vi "EPTx_RT_mul-inj_Final.vi"(0 "EPTxSupervisor_rt":T13={"Sync"=FALSE, "CurrentCAD"=0.0, "MaxCAD"=720.0, "HistoryCAD"=61.0, "CADRate"=0.0, "AvgSpeed"=0.0, "Config"=FALSE, "Rcvg Primary"=FALSE, "Stall"=FALSE, "Overflow"=FALSE, "Ratio Error"=FALSE, "Pattern Error"=FALSE, "Aux Warning"=FALSE, "Watchdog Error"=FALSE}, 1 "PatternConfig":T16 {"Max Rate [Hz]" format="%#_3p"}, 2 "SimulatorConfig":T18={"Sim Speed [RPM]"=1000.0, "Ramp Rate [RPM/s]"=50.0, "Rotations"=2, "Pause"=FALSE, "Pause Angle [CAD]"=0.0, "Max Offset [RPM]"=0.0, "Cylinders"=6}, 5 "EPTxState":T15={"Sync Enable"=TRUE, "Clear Errors"=FALSE, "Sim Enable"=FALSE, "Sim Speed [RPM]"=1000.0}, 7 "EPTxFilters":T14={"Primary [s]"=5e-06, "Aux 1 [s]"=5e-06, "Aux 2 [s]"=0.0, "Aux 3 [s]"=0.0, "Aux 4 [s]"=0.0} {"Aux 4 [s]" format="%#_6p"; "Aux 3 [s]" format="%#_6p"; "Aux 2 [s]" format="%#_6p"; "Aux 1 [s]" format="%#_6p"; "Primary [s]" format="%#_6p"}, 9 "RT_Input":T17={"Load"=FALSE, "History_[CAD]"=63, "Stall_Speed_[RPM]"=200.0, "Delay_time[ms]"=0.0, "DrvMode"=0} caption="簇", 11 "Inj_Timing":T12, 12 "Inj_Duration_in":T11) -> (3 "Config_number":T10 caption="簇", 4 "CylinderSig":T6={"CylinderSig_1"={"Cylinder1_H_R[CAD]"=204.0, "Cylinder1_H_F[CAD]"=210.0}, "CylinderSig_2"={"Cylinder2_H_R[CAD]"=684.0, "Cylinder2_H_F[CAD]"=690.0}, "CylinderSig_3"={"Cylinder3_H_R[CAD]"=444.0, "Cylinder3_H_F[CAD]"=450.0}, "CylinderSig_4"={"Cylinder4_H_R[CAD]"=90.0, "Cylinder4_H_F[CAD]"=100.0}, "CylinderSig_5"={"Cylinder5_H_R[CAD]"=324.0, "Cylinder5_H_F[CAD]"=330.0}, "CylinderSig_6"={"Cylinder6_H_R[CAD]"=0.0, "Cylinder6_H_F[CAD]"=0.0}} caption="簇", 6 "EPTxPatternConfig":T4 {"Pattern"."Aux 4" format="%#_16g"; "Pattern"."Aux 3" format="%#_16g"; "Pattern"."Aux 2" format="%#_16g"; "Pattern"."Aux 1" format="%#_16g"; "Pattern"."Primary" format="%#_16g"}, 8 "Tick_output":T1, 10 "EPTxControl":T3={"Sync Enable"=FALSE, "Clear Errors"=FALSE, "Sim Enable"=FALSE, "Sim Rate"=63.999996185302734, "Watchdog"=FALSE}, 13 "Cmd_Seq":T19, 14 "Lighting":T7 caption="簇", 15 "EPTxData":T2={"Sync"=TRUE, "CurrentCAD"=122.91406, "Speed [RPM]"=999.75, "Config"=FALSE, "Rcvg Primary"=TRUE, "Stall"=FALSE, "Overflow"=FALSE, "Ratio Error"=FALSE, "Pattern Error"=FALSE, "Aux Warning"=FALSE, "Watchdog Error"=FALSE})   [LabVIEW 2023]
uses:
  <vilib>/Powertrain Controls/Device Drivers/Engine Position Tracking/EPTx/RevA/RT/Controls/Simulator Config.ctl
  <vilib>/Powertrain Controls/Device Drivers/Engine Position Tracking/EPTx/RevA/RT/Controls/Pattern Config.ctl
  <vilib>/Powertrain Controls/Device Drivers/Engine Position Tracking/EPTx/RevA/RT/Controls/EPTxState.ctl
  <vilib>/Powertrain Controls/Device Drivers/Engine Position Tracking/EPTx/RevA/RT/Controls/EPTxFilters.ctl
  <vilib>/Powertrain Controls/Device Drivers/Engine Position Tracking/EPTx/RevA/FPGA/Controls/EPTxSupervisor.ctl
  <vilib>/Powertrain Controls/Device Drivers/Engine Position Tracking/EPTx/RevA/FPGA/Controls/EPTxConfig.ctl
  <vilib>/Powertrain Controls/Device Drivers/Engine Position Tracking/EPTx/RevA/FPGA/Controls/EPTxSimulatorConfig.ctl
  <vilib>/Powertrain Controls/Device Drivers/Engine Position Tracking/EPTx/RevA/FPGA/Controls/EPTxPatternConfig.ctl
  <vilib>/Powertrain Controls/Device Drivers/Engine Position Tracking/EPTx/RevA/FPGA/Controls/Patterns.ctl
  <vilib>/Powertrain Controls/Device Drivers/Engine Position Tracking/EPTx/RevA/FPGA/Controls/EPTxControl.ctl
  <vilib>/Powertrain Controls/Device Drivers/Engine Position Tracking/EPTx/RevA/RT/Controls/EPTxData.ctl
  <vilib>/Powertrain Controls/Device Drivers/Engine Position Tracking/EPTx/RevA/RT/Controls/EPTxPattern.ctl
  <vilib>/Powertrain Controls/Device Drivers/Engine Position Tracking/EPTx/RevA/RT/Controls/Pattern.ctl
  <vilib>/Powertrain Controls/Device Drivers/Engine Position Tracking/EPTx/RevA/RT/Controls/EPTxSettings.ctl
  <vilib>/Powertrain Controls/Device Drivers/Engine Position Tracking/EPTx/RevA/RT/Controls/Settings - Tooth.ctl
  <vilib>/Powertrain Controls/Device Drivers/Engine Position Tracking/EPTx/RevA/RT/Controls/Direction Detection.ctl
  <vilib>/Powertrain Controls/Device Drivers/Engine Position Tracking/EPTx/RevA/RT/Controls/Settings - Pattern.ctl
  <vilib>/Powertrain Controls/Device Drivers/Engine Position Tracking/EPTx/RevA/RT/Controls/Settings - Token.ctl
  <vilib>/Powertrain Controls/Device Drivers/Engine Position Tracking/EPTx/RevA/RT/Controls/Aux Signal.ctl
  <vilib>/Powertrain Controls/Device Drivers/Engine Position Tracking/EPTx/RevA/RT/Controls/Aux Type.ctl
  <vilib>/Powertrain Controls/Device Drivers/Engine Position Tracking/EPTx/RevA/RT/Controls/Aux Threshold.ctl
  <vilib>/Powertrain Controls/Device Drivers/Engine Position Tracking/EPTx/RevA/RT/EPTx - RevA - RT.lvlib
  <vilib>/Powertrain Controls/Device Drivers/Engine Position Tracking/EPTx/RevA/FPGA/EPTx - RevA - FPGA.lvlib
panel:
  out "CAD":sgl
  out "AvgSpeed":fxp<+,17,15>
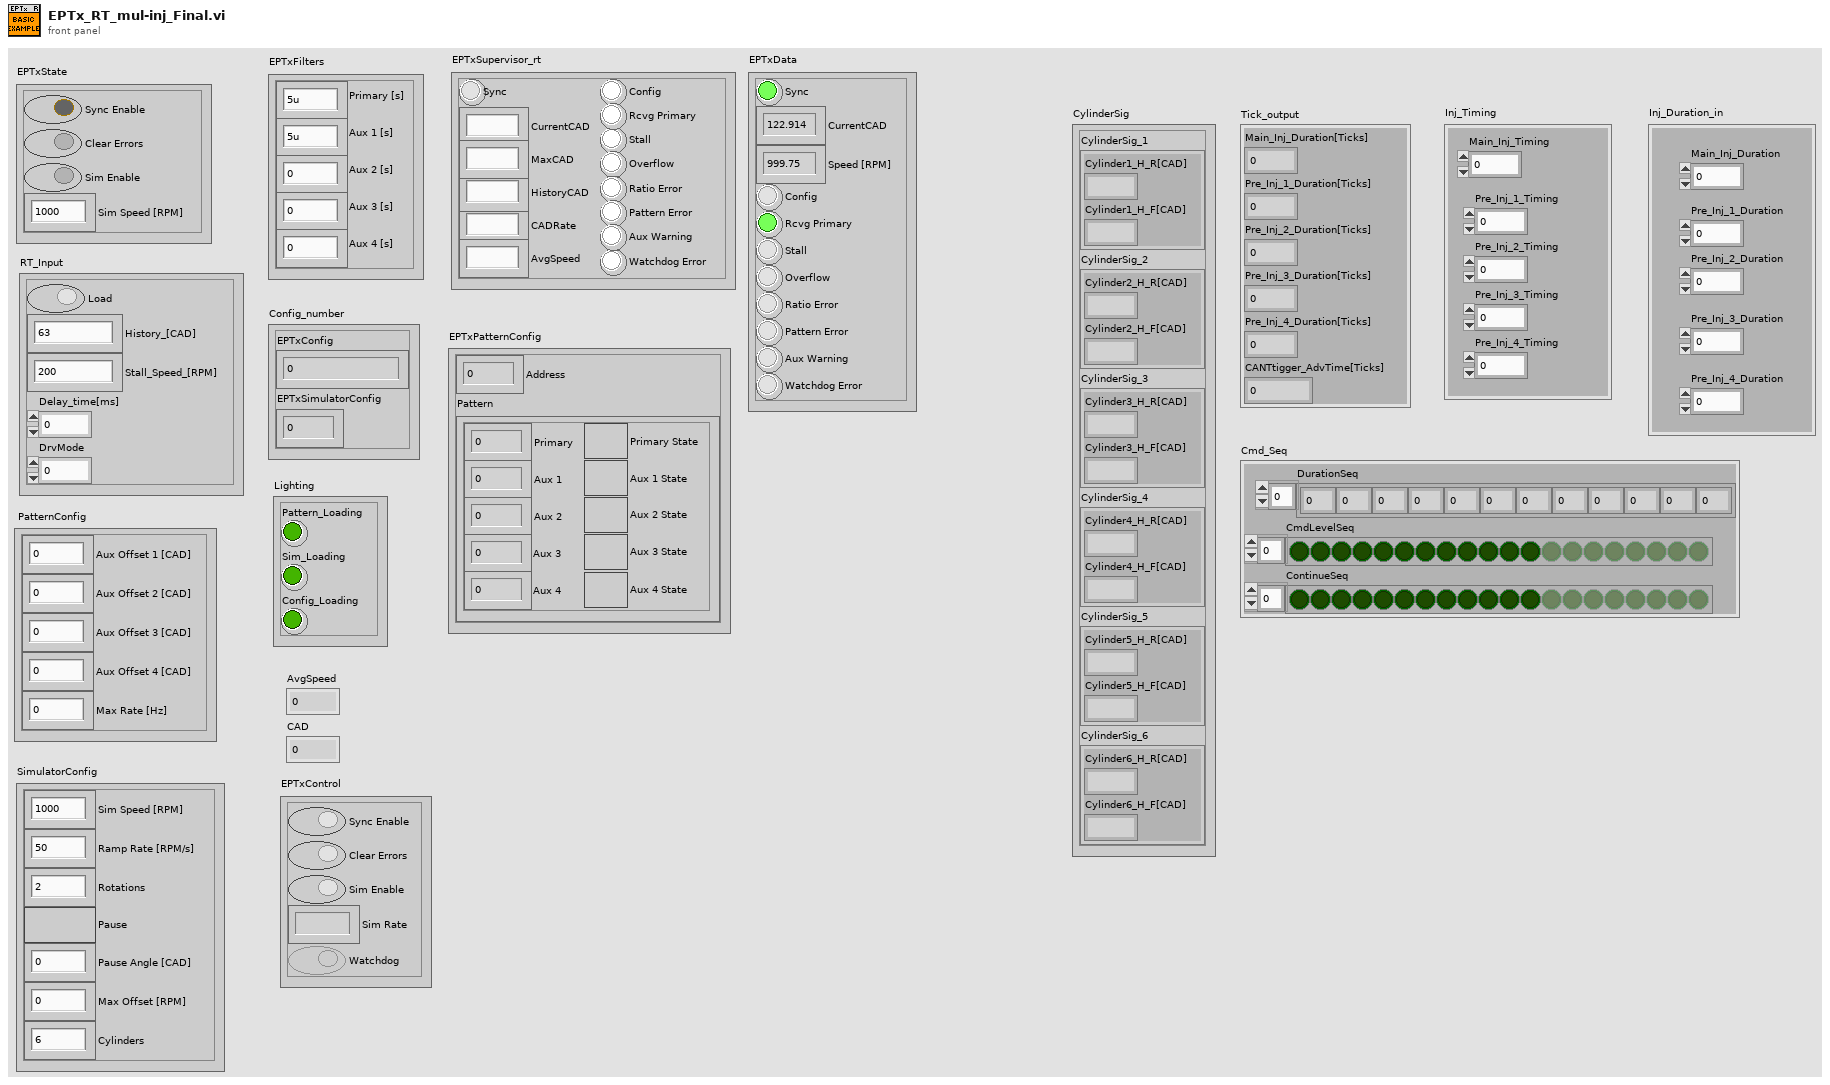
[diagram p1: front panel]
types:
  T1 = cluster{"Main_Inj_Duration[Ticks]":u32, "Pre_Inj_1_Duration[Ticks]":u32, "Pre_Inj_2_Duration[Ticks]":u32, "Pre_Inj_3_Duration[Ticks]":u32, "Pre_Inj_4_Duration[Ticks]":u32, "CANTtigger_AdvTime[Ticks]":u32}
  T2 = typedef "EPTx - RevA - RT.lvlib/EPTxData.ctl" = cluster{"Sync":bool, "CurrentCAD":sgl, "Speed [RPM]":sgl, "Config":bool, "Rcvg Primary":bool, "Stall":bool, "Overflow":bool, "Ratio Error":bool, "Pattern Error":bool, "Aux Warning":bool, "Watchdog Error":bool}
  T3 = typedef "EPTx - RevA - FPGA.lvlib/EPTxControl.ctl" = cluster{"Sync Enable":bool, "Clear Errors":bool, "Sim Enable":bool, "Sim Rate":fxp<+,24,6>, "Watchdog":bool}
  T4 = typedef "EPTx - RevA - FPGA.lvlib/EPTxPatternConfig.ctl" = cluster{"Address":fxp<+,14,14>, "Pattern":T5}
  T5 = typedef "EPTx - RevA - FPGA.lvlib/Patterns.ctl" = cluster{"Primary":fxp<+,19,12>, "Primary State":bool, "Aux 1":fxp<+,19,12>, "Aux 1 State":bool, "Aux 2":fxp<+,19,12>, "Aux 2 State":bool, "Aux 3":fxp<+,19,12>, "Aux 3 State":bool, "Aux 4":fxp<+,19,12>, "Aux 4 State":bool}
  T6 = cluster{"CylinderSig_1":cluster{"Cylinder1_H_R[CAD]":fxp<+,18,11>, "Cylinder1_H_F[CAD]":fxp<+,18,11>}, "CylinderSig_2":cluster{"Cylinder2_H_R[CAD]":fxp<+,18,11>, "Cylinder2_H_F[CAD]":fxp<+,18,11>}, "CylinderSig_3":cluster{"Cylinder3_H_R[CAD]":fxp<+,18,11>, "Cylinder3_H_F[CAD]":fxp<+,18,11>}, "CylinderSig_4":cluster{"Cylinder4_H_R[CAD]":fxp<+,18,11>, "Cylinder4_H_F[CAD]":fxp<+,18,11>}, "CylinderSig_5":cluster{"Cylinder5_H_R[CAD]":fxp<+,18,11>, "Cylinder5_H_F[CAD]":fxp<+,18,11>}, "CylinderSig_6":cluster{"Cylinder6_H_R[CAD]":fxp<+,18,11>, "Cylinder6_H_F[CAD]":fxp<+,18,11>}}
  T7 = cluster{"Pattern_Loading":bool, "Sim_Loading":bool, "Config_Loading":bool}
  T8 = typedef "EPTx - RevA - FPGA.lvlib/EPTxConfig.ctl" = u64
  T9 = typedef "EPTx - RevA - FPGA.lvlib/EPTxSimulatorConfig.ctl" = u32
  T10 = cluster{"EPTxConfig":T8, "EPTxSimulatorConfig":T9}
  T11 = cluster{"Main_Inj_Duration":sgl, "Pre_Inj_1_Duration":sgl, "Pre_Inj_2_Duration":sgl, "Pre_Inj_3_Duration":sgl, "Pre_Inj_4_Duration":sgl}
  T12 = cluster{"Main_Inj_Timing":sgl, "Pre_Inj_1_Timing":sgl, "Pre_Inj_2_Timing":sgl, "Pre_Inj_3_Timing":sgl, "Pre_Inj_4_Timing":sgl}
  T13 = typedef "EPTx - RevA - FPGA.lvlib/EPTxSupervisor.ctl" = cluster{"Sync":bool, "CurrentCAD":fxp<+,18,11>, "MaxCAD":fxp<+,11,11>, "HistoryCAD":fxp<+,11,11>, "CADRate":fxp<+,22,8>, "AvgSpeed":fxp<+,17,15>, "Config":bool, "Rcvg Primary":bool, "Stall":bool, "Overflow":bool, "Ratio Error":bool, "Pattern Error":bool, "Aux Warning":bool, "Watchdog Error":bool}
  T14 = typedef "EPTx - RevA - RT.lvlib/EPTxFilters.ctl" = cluster{"Primary [s]":sgl, "Aux 1 [s]":sgl, "Aux 2 [s]":sgl, "Aux 3 [s]":sgl, "Aux 4 [s]":sgl}
  T15 = typedef "EPTx - RevA - RT.lvlib/EPTxState.ctl" = cluster{"Sync Enable":bool, "Clear Errors":bool, "Sim Enable":bool, "Sim Speed [RPM]":sgl}
  T16 = typedef "EPTx - RevA - RT.lvlib/Pattern Config.ctl" = cluster{"Aux Offset 1 [CAD]":sgl, "Aux Offset 2 [CAD]":sgl, "Aux Offset 3 [CAD]":sgl, "Aux Offset 4 [CAD]":sgl, "Max Rate [Hz]":sgl}
  T17 = cluster{"Load":bool, "History_[CAD]":u8, "Stall_Speed_[RPM]":sgl, "Delay_time[ms]":sgl, "DrvMode":u32}
  T18 = typedef "EPTx - RevA - RT.lvlib/Simulator Config.ctl" = cluster{"Sim Speed [RPM]":sgl, "Ramp Rate [RPM/s]":sgl, "Rotations":u8, "Pause":bool, "Pause Angle [CAD]":sgl, "Max Offset [RPM]":sgl, "Cylinders":u8}
  T19 = cluster{"DurationSeq":u32[], "CmdLevelSeq":bool[], "ContinueSeq":bool[]}
  T20 = cluster{"Duration1":sgl, "Duratiion2":sgl, "Duration3":sgl, "Duration4":sgl, "Duration5":sgl, "Duration6":sgl, "Duration7":sgl, "Duration8":sgl, "Duration9":sgl, "Duration10":sgl, "Duration11":sgl, "Duration12":sgl}
  T21 = cluster{"CylinderSig_1":cluster{"Cylinder1_H_R [CAD]":fxp<+,18,11>, "Cylinder1_H_F [CAD]":fxp<+,18,11>}, "CylinderSig_2":cluster{"Cylinder2_H_R [CAD]":fxp<+,18,11>, "Cylinder2_H_F [CAD]":fxp<+,18,11>}, "CylinderSig_3":cluster{"Cylinder3_H_R [CAD]":fxp<+,18,11>, "Cylinder3_H_F [CAD]":fxp<+,18,11>}, "CylinderSig_4":cluster{"Cylinder4_H_R [CAD]":fxp<+,18,11>, "Cylinder4_H_F [CAD]":fxp<+,18,11>}, "CylinderSig_5":cluster{"Cylinder5_H_R [CAD]":fxp<+,18,11>, "Cylinder5_H_F [CAD]":fxp<+,18,11>}, "CylinderSig_6":cluster{"Cylinder6_H_R [CAD]":fxp<+,18,11>, "Cylinder6_H_F [CAD]":fxp<+,18,11>}}
  T22 = cluster{"Cylinder6_H_R [CAD]":fxp<+,18,11>, "Cylinder6_H_F [CAD]":fxp<+,18,11>}
  T23 = cluster{"Cylinder5_H_R [CAD]":fxp<+,18,11>, "Cylinder5_H_F [CAD]":fxp<+,18,11>}
  T24 = cluster{"Cylinder4_H_R [CAD]":fxp<+,18,11>, "Cylinder4_H_F [CAD]":fxp<+,18,11>}
  T25 = cluster{"Cylinder3_H_R [CAD]":fxp<+,18,11>, "Cylinder3_H_F [CAD]":fxp<+,18,11>}
  T26 = cluster{"Cylinder2_H_R [CAD]":fxp<+,18,11>, "Cylinder2_H_F [CAD]":fxp<+,18,11>}
  T27 = cluster{"Cylinder1_H_R [CAD]":fxp<+,18,11>, "Cylinder1_H_F [CAD]":fxp<+,18,11>}
  T28 = cluster{"Pattern Loading":bool, "Sim Loading":bool, "Config Loading":bool}
  T29 = typedef "EPTx - RevA - RT.lvlib/EPTxSettings.ctl" = cluster{"Rotation":u8, "Ratios":sgl[], "Thresholds":sgl[], "Tooth":T30, "Pattern":T32[], "Token":T33[], "Aux Threshold Min":T36, "Aux Threshold Max":T36}
  T30 = typedef "EPTx - RevA - RT.lvlib/Settings - Tooth.ctl" = cluster{"Rising Edge":bool, "Falling Edge":bool, "Direction\nDetection":T31, "Level":bool, "Parameter":sgl}
  T31 = typedef "EPTx - RevA - RT.lvlib/Direction Detection.ctl" = enum16{"None", "Aux Signal", "Length"}
  T32 = typedef "EPTx - RevA - RT.lvlib/Settings - Pattern.ctl" = cluster{"Ratio Index":u8, "Ratio Count":u16, "Angle":sgl, "dAngle":sgl}
  T33 = typedef "EPTx - RevA - RT.lvlib/Settings - Token.ctl" = cluster{"Length":u16, "Start Index":u8, "Start Count":u16, "Aux 1":T34, "Aux 1 Type":T35, "Aux 1 Max":u16, "Aux 1 Min":u16, "Aux 2":T34, "Aux 2 Type":T35, "Aux 2 Max":u16, "Aux 2 Min":u16, "End Index":u8, "End Count":u16}
  T34 = typedef "EPTx - RevA - RT.lvlib/Aux Signal.ctl" = enum8{"---", "Aux 1", "Aux 2", "Aux 3", "Aux 4"}
  T35 = typedef "EPTx - RevA - RT.lvlib/Aux Type.ctl" = enum8{"Falling", "Rising", "Low", "High", "Ratio"}
  T36 = typedef "EPTx - RevA - RT.lvlib/Aux Threshold.ctl" = cluster{"Aux 1":sgl, "Aux 2":sgl, "Aux 3":sgl, "Aux 4":sgl}
  T37 = typedef "EPTx - RevA - RT.lvlib/EPTxPattern.ctl" = cluster{"Rotations":u8, "Cylinders":u8, "Primary":T38[], "Aux 1":T38[], "Aux 2":T38[], "Aux 3":T38[], "Aux 4":T38[]}
  T38 = typedef "EPTx - RevA - RT.lvlib/Pattern.ctl" = cluster{"Angle":sgl, "State":bool}
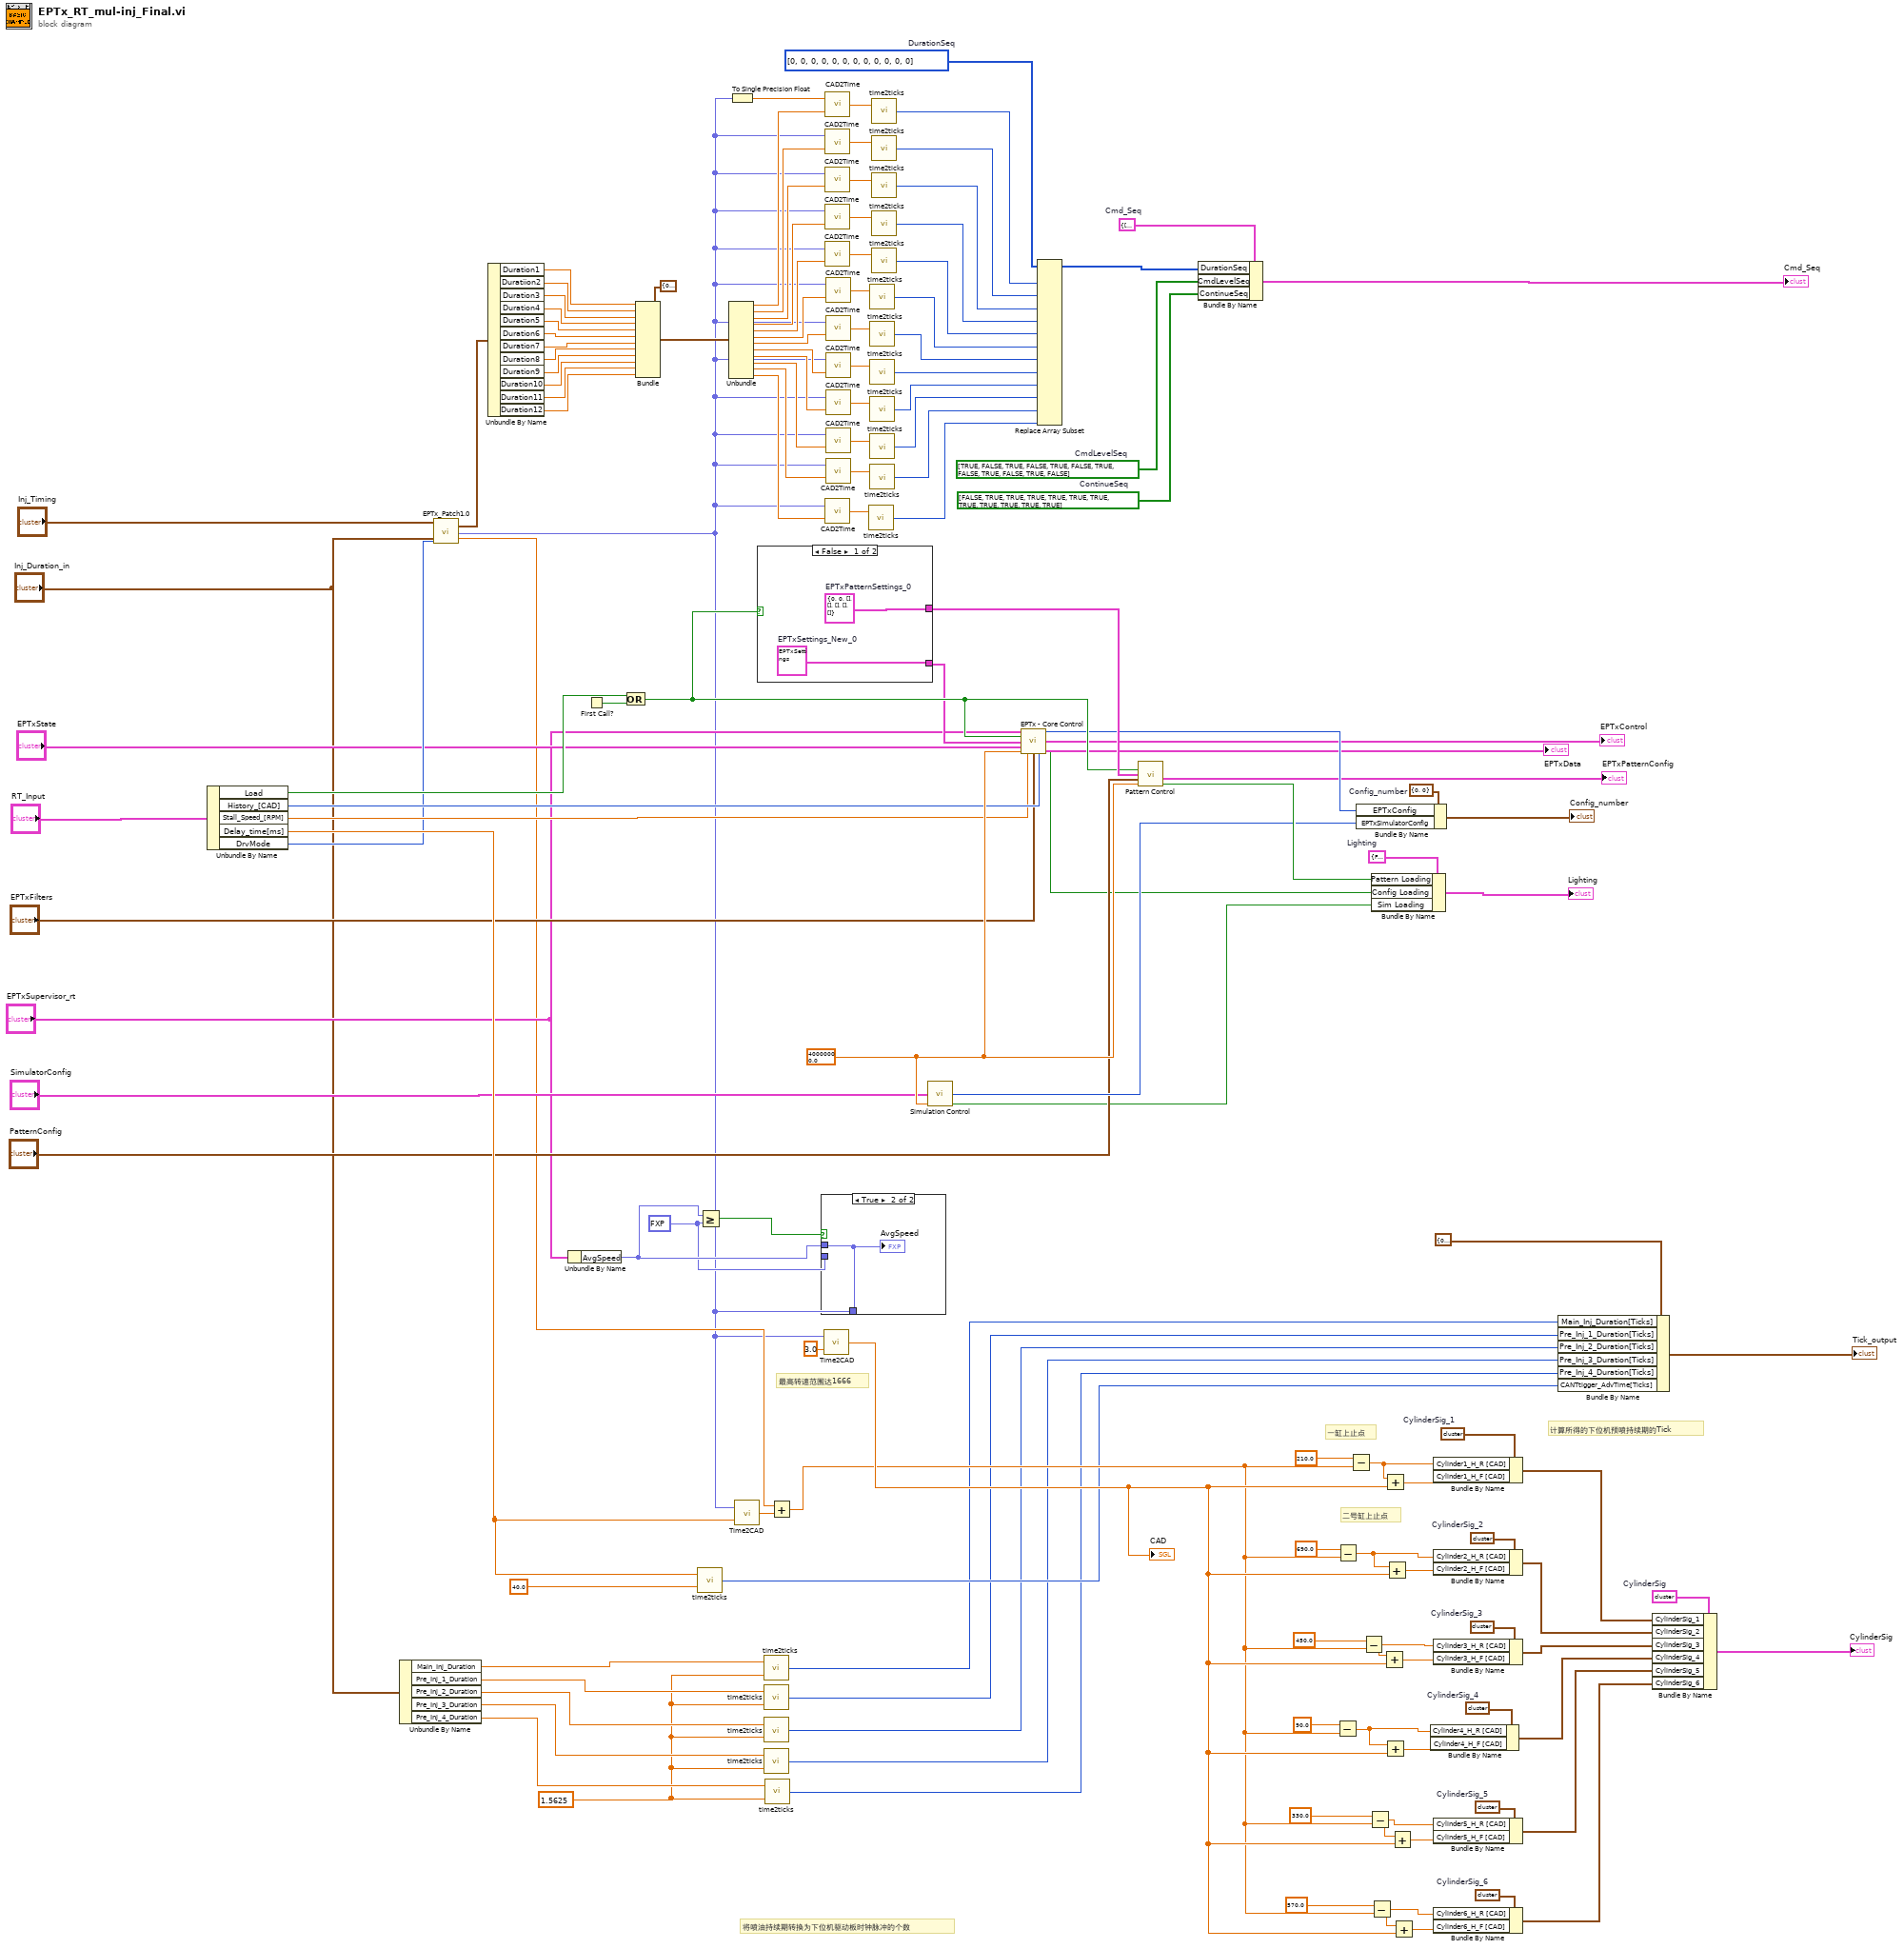
[diagram p0: block diagram]
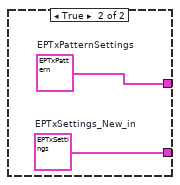
[diagram p3: hidden frame]
diagram:
  w6 = bool[] [TRUE, FALSE, TRUE, FALSE, TRUE, FALSE, TRUE, FALSE, TRUE, FALSE, TRUE, FALSE]  # CmdLevelSeq
  w7 = bool[] [FALSE, TRUE, TRUE, TRUE, TRUE, TRUE, TRUE, TRUE, TRUE, TRUE, TRUE, TRUE]  # ContinueSeq
  w8 = fxp<+,7,8> 250.0 ("y")
  w96 = T19 {"DurationSeq"=[0, 0, 0, 0, 0, 0, 0, 0, 0, 0, 0, 0], "CmdLevelSeq"=[FALSE, FALSE, FALSE, FALSE, FALSE, FALSE, FALSE, FALSE, FALSE, FALSE, FALSE, FALSE], "ContinueSeq"=[FALSE, FALSE, FALSE, FALSE, FALSE, FALSE, FALSE, FALSE, FALSE, FALSE, FALSE, FALSE]}  # Cmd_Seq
  w80 = u32[] [0, 0, 0, 0, 0, 0, 0, 0, 0, 0, 0, 0]  # DurationSeq
  w10 = sgl 1.5625 ("y")
  w111 = T21 {"CylinderSig_1"={"Cylinder1_H_R [CAD]"=204.0, "Cylinder1_H_F [CAD]"=210.0}, "CylinderSig_2"={"Cylinder2_H_R [CAD]"=684.0, "Cylinder2_H_F [CAD]"=690.0}, "CylinderSig_3"={"Cylinder3_H_R [CAD]"=444.0, "Cylinder3_H_F [CAD]"=450.0}, "CylinderSig_4"={"Cylinder4_H_R [CAD]"=90.0, "Cylinder4_H_F [CAD]"=100.0}, "CylinderSig_5"={"Cylinder5_H_R [CAD]"=324.0, "Cylinder5_H_F [CAD]"=330.0}, "CylinderSig_6"={"Cylinder6_H_R [CAD]"=0.0, "Cylinder6_H_F [CAD]"=0.0}}  # CylinderSig
  w128 = T22 {"Cylinder6_H_R [CAD]"=0.0, "Cylinder6_H_F [CAD]"=0.0}  # CylinderSig_6
  w129 = T23 {"Cylinder5_H_R [CAD]"=324.0, "Cylinder5_H_F [CAD]"=330.0}  # CylinderSig_5
  w130 = T24 {"Cylinder4_H_R [CAD]"=90.0, "Cylinder4_H_F [CAD]"=100.0}  # CylinderSig_4
  w131 = T25 {"Cylinder3_H_R [CAD]"=444.0, "Cylinder3_H_F [CAD]"=450.0}  # CylinderSig_3
  w132 = T26 {"Cylinder2_H_R [CAD]"=684.0, "Cylinder2_H_F [CAD]"=690.0}  # CylinderSig_2
  w133 = T27 {"Cylinder1_H_R [CAD]"=204.0, "Cylinder1_H_F [CAD]"=210.0}  # CylinderSig_1
  w138 = T10 {"EPTxConfig"=0, "EPTxSimulatorConfig"=0}  # Config_number
  w140 = T28 {"Pattern Loading"=FALSE, "Sim Loading"=FALSE, "Config Loading"=FALSE}  # Lighting
  w144 = sgl 40000000.0 ("Frequency (40M) [Hz]")
  # "最高转速范围达1666"
  # "计算所得的下位机预喷持续期的Tick"
  # "二号缸上止点"
  # "一缸上止点"
  # "将喷油持续期转换为下位机驱动板时钟脉冲的个数"
  n1 = Unbundle By Name("RT_Input") -> ("Load"=w136:bool, "History_[CAD]"=w135:u8, "Stall_Speed_[RPM]"=w134:sgl, "Delay_time[ms]"=w98:sgl, "DrvMode"=w28:u32)
  n2 = Unbundle By Name("Inj_Duration_in") -> ("Main_Inj_Duration"=w36:sgl, "Pre_Inj_1_Duration"=w35:sgl, "Pre_Inj_2_Duration"=w34:sgl, "Pre_Inj_3_Duration"=w33:sgl, "Pre_Inj_4_Duration"=w32:sgl)
  n3 = Unbundle By Name("EPTxSupervisor_rt") -> ("AvgSpeed"=w15:fxp<+,17,15>)
  n4 = First Call?() -> (First Call?: T/F=w142:bool)
  n5 = Compound Arithmetic op=OR ("复合运算")(w136, w142) -> (w141:bool)
  n6 = call <vilib>:"time2ticks.vi"("Clock Frequency (MHz, 40)"=sgl 40.0, "Time (msec)"=w98) -> ("Ticks"=w42:u32)
  n7 = Greater Or Equal?(x=w15, y=w8) -> (x >= y?=w16:bool)
  n8 = case shown="False" w141 {
    tunnel: [w146 w148] -> w143
    tunnel: [w145 w147] -> w101
    frame False {
      w145 = T29 {"Rotation"=0, "Ratios"=[], "Thresholds"=[], "Tooth"={"Rising Edge"=FALSE, "Falling Edge"=FALSE, "Direction\nDetection"=enum."None", "Level"=FALSE, "Parameter"=0.0}, "Pattern"=[], "Token"=[], "Aux Threshold Min"={"Aux 1"=0.0, "Aux 2"=0.0, "Aux 3"=0.0, "Aux 4"=0.0}, "Aux Threshold Max"={"Aux 1"=0.0, "Aux 2"=0.0, "Aux 3"=0.0, "Aux 4"=0.0}}  # EPTxSettings_New_0
      w146 = T37 {"Rotations"=0, "Cylinders"=0, "Primary"=[], "Aux 1"=[], "Aux 2"=[], "Aux 3"=[], "Aux 4"=[]}  # EPTxPatternSettings_0
    }
    frame True {
      w147 = T29 {"Rotation"=2, "Ratios"=[0.33333334, 1.0, 3.0], "Thresholds"=[0.16666667, 0.6666667, 0.6666667, 2.0, 2.0, 4.0, 999.0], "Tooth"={"Rising Edge"=TRUE, "Falling Edge"=FALSE, "Direction\nDetection"=enum."None", "Level"=FALSE, "Parameter"=0.0}, "Pattern"=[{"Ratio Index"=0, "Ratio Count"=1, "Angle"=0.0, "dAngle"=6.0}, {"Ratio Index"=1, "Ratio Count"=56, "Angle"=6.0, "dAngle"=6.0}, {"Ratio Index"=2, "Ratio Count"=1, "Angle"=342.0, "dAngle"=18.0}, {"Ratio Index"=0, "Ratio Count"=1, "Angle"=360.0, "dAngle"=6.0}, {"Ratio Index"=1, "Ratio Count"=56, "Angle"=366.0, "dAngle"=6.0}, {"Ratio Index"=2, "Ratio Count"=1, "Angle"=702.0, "dAngle"=18.0}], "Token"=[{"Length"=1, "Start Index"=5, "Start Count"=0, "Aux 1"=enum."---", "Aux 1 Type"=enum."Falling", "Aux 1 Max"=0, "Aux 1 Min"=0, "Aux 2"=enum."Aux 2", "Aux 2 Type"=enum."Ratio", "Aux 2 Max"=73, "Aux 2 Min"=73, "End Index"=0, "End Count"=0}], "Aux Threshold Min"={"Aux 1"=1.8809524, "Aux 2"=1.2142857, "Aux 3"=0.0, "Aux 4"=0.0}, "Aux Threshold Max"={"Aux 1"=2.7857144, "Aux 2"=1.8809524, "Aux 3"=999.0, "Aux 4"=999.0}}  # EPTxSettings_New_in
      w148 = T37 {"Rotations"=2, "Cylinders"=6, "Primary"=[{"Angle"=0.0, "State"=FALSE}, {"Angle"=3.0, "State"=TRUE}, {"Angle"=6.0, "State"=FALSE}, {"Angle"=9.0, "State"=TRUE}, {"Angle"=12.0, "State"=FALSE}, {"Angle"=15.0, "State"=TRUE}, {"Angle"=18.0, "State"=FALSE}, {"Angle"=21.0, "State"=TRUE}, {"Angle"=24.0, "State"=FALSE}, {"Angle"=27.0, "State"=TRUE}, {"Angle"=30.0, "State"=FALSE}, {"Angle"=33.0, "State"=TRUE}, {"Angle"=36.0, "State"=FALSE}, {"Angle"=39.0, "State"=TRUE}, {"Angle"=42.0, "State"=FALSE}, {"Angle"=45.0, "State"=TRUE}, {"Angle"=48.0, "State"=FALSE}, {"Angle"=51.0, "State"=TRUE}, {"Angle"=54.0, "State"=FALSE}, {"Angle"=57.0, "State"=TRUE}, {"Angle"=60.0, "State"=FALSE}, {"Angle"=63.0, "State"=TRUE}, {"Angle"=66.0, "State"=FALSE}, {"Angle"=69.0, "State"=TRUE}, {"Angle"=72.0, "State"=FALSE}, {"Angle"=75.0, "State"=TRUE}, {"Angle"=78.0, "State"=FALSE}, {"Angle"=81.0, "State"=TRUE}, {"Angle"=84.0, "State"=FALSE}, {"Angle"=87.0, "State"=TRUE}, {"Angle"=90.0, "State"=FALSE}, {"Angle"=93.0, "State"=TRUE}, {"Angle"=96.0, "State"=FALSE}, {"Angle"=99.0, "State"=TRUE}, {"Angle"=102.0, "State"=FALSE}, {"Angle"=105.0, "State"=TRUE}, {"Angle"=108.0, "State"=FALSE}, {"Angle"=111.0, "State"=TRUE}, {"Angle"=114.0, "State"=FALSE}, {"Angle"=117.0, "State"=TRUE}, {"Angle"=120.0, "State"=FALSE}, {"Angle"=123.0, "State"=TRUE}, {"Angle"=126.0, "State"=FALSE}, {"Angle"=129.0, "State"=TRUE}, {"Angle"=132.0, "State"=FALSE}, {"Angle"=135.0, "State"=TRUE}, {"Angle"=138.0, "State"=FALSE}, {"Angle"=141.0, "State"=TRUE}, {"Angle"=144.0, "State"=FALSE}, {"Angle"=147.0, "State"=TRUE}, {"Angle"=150.0, "State"=FALSE}, {"Angle"=153.0, "State"=TRUE}, {"Angle"=156.0, "State"=FALSE}, {"Angle"=159.0, "State"=TRUE}, {"Angle"=162.0, "State"=FALSE}, {"Angle"=165.0, "State"=TRUE}, {"Angle"=168.0, "State"=FALSE}, {"Angle"=171.0, "State"=TRUE}, {"Angle"=174.0, "State"=FALSE}, {"Angle"=177.0, "State"=TRUE}, {"Angle"=180.0, "State"=FALSE}, {"Angle"=183.0, "State"=TRUE}, {"Angle"=186.0, "State"=FALSE}, {"Angle"=189.0, "State"=TRUE}, {"Angle"=192.0, "State"=FALSE}, {"Angle"=195.0, "State"=TRUE}, {"Angle"=198.0, "State"=FALSE}, {"Angle"=201.0, "State"=TRUE}, {"Angle"=204.0, "State"=FALSE}, {"Angle"=207.0, "State"=TRUE}, {"Angle"=210.0, "State"=FALSE}, {"Angle"=213.0, "State"=TRUE}, {"Angle"=216.0, "State"=FALSE}, {"Angle"=219.0, "State"=TRUE}, {"Angle"=222.0, "State"=FALSE}, {"Angle"=225.0, "State"=TRUE}, {"Angle"=228.0, "State"=FALSE}, {"Angle"=231.0, "State"=TRUE}, {"Angle"=234.0, "State"=FALSE}, {"Angle"=237.0, "State"=TRUE}, {"Angle"=240.0, "State"=FALSE}, {"Angle"=243.0, "State"=TRUE}, {"Angle"=246.0, "State"=FALSE}, {"Angle"=249.0, "State"=TRUE}, {"Angle"=252.0, "State"=FALSE}, {"Angle"=255.0, "State"=TRUE}, {"Angle"=258.0, "State"=FALSE}, {"Angle"=261.0, "State"=TRUE}, {"Angle"=264.0, "State"=FALSE}, {"Angle"=267.0, "State"=TRUE}, {"Angle"=270.0, "State"=FALSE}, {"Angle"=273.0, "State"=TRUE}, {"Angle"=276.0, "State"=FALSE}, {"Angle"=279.0, "State"=TRUE}, {"Angle"=282.0, "State"=FALSE}, {"Angle"=285.0, "State"=TRUE}, {"Angle"=288.0, "State"=FALSE}, {"Angle"=291.0, "State"=TRUE}, {"Angle"=294.0, "State"=FALSE}, {"Angle"=297.0, "State"=TRUE}, {"Angle"=300.0, "State"=FALSE}, {"Angle"=303.0, "State"=TRUE}, {"Angle"=306.0, "State"=FALSE}, {"Angle"=309.0, "State"=TRUE}, {"Angle"=312.0, "State"=FALSE}, {"Angle"=315.0, "State"=TRUE}, {"Angle"=318.0, "State"=FALSE}, {"Angle"=321.0, "State"=TRUE}, {"Angle"=324.0, "State"=FALSE}, {"Angle"=327.0, "State"=TRUE}, {"Angle"=330.0, "State"=FALSE}, {"Angle"=333.0, "State"=TRUE}, {"Angle"=336.0, "State"=FALSE}, {"Angle"=339.0, "State"=TRUE}, {"Angle"=342.0, "State"=FALSE}, {"Angle"=345.0, "State"=TRUE}, {"Angle"=360.0, "State"=FALSE}, {"Angle"=363.0, "State"=TRUE}, {"Angle"=366.0, "State"=FALSE}, {"Angle"=369.0, "State"=TRUE}, {"Angle"=372.0, "State"=FALSE}, {"Angle"=375.0, "State"=TRUE}, {"Angle"=378.0, "State"=FALSE}, {"Angle"=381.0, "State"=TRUE}, {"Angle"=384.0, "State"=FALSE}, {"Angle"=387.0, "State"=TRUE}, {"Angle"=390.0, "State"=FALSE}, {"Angle"=393.0, "State"=TRUE}, {"Angle"=396.0, "State"=FALSE}, {"Angle"=399.0, "State"=TRUE}, {"Angle"=402.0, "State"=FALSE}, {"Angle"=405.0, "State"=TRUE}, {"Angle"=408.0, "State"=FALSE}, {"Angle"=411.0, "State"=TRUE}, {"Angle"=414.0, "State"=FALSE}, {"Angle"=417.0, "State"=TRUE}, {"Angle"=420.0, "State"=FALSE}, {"Angle"=423.0, "State"=TRUE}, {"Angle"=426.0, "State"=FALSE}, {"Angle"=429.0, "State"=TRUE}, {"Angle"=432.0, "State"=FALSE}, {"Angle"=435.0, "State"=TRUE}, {"Angle"=438.0, "State"=FALSE}, {"Angle"=441.0, "State"=TRUE}, {"Angle"=444.0, "State"=FALSE}, {"Angle"=447.0, "State"=TRUE}, {"Angle"=450.0, "State"=FALSE}, {"Angle"=453.0, "State"=TRUE}, {"Angle"=456.0, "State"=FALSE}, {"Angle"=459.0, "State"=TRUE}, {"Angle"=462.0, "State"=FALSE}, {"Angle"=465.0, "State"=TRUE}, {"Angle"=468.0, "State"=FALSE}, {"Angle"=471.0, "State"=TRUE}, {"Angle"=474.0, "State"=FALSE}, {"Angle"=477.0, "State"=TRUE}, {"Angle"=480.0, "State"=FALSE}, {"Angle"=483.0, "State"=TRUE}, {"Angle"=486.0, "State"=FALSE}, {"Angle"=489.0, "State"=TRUE}, {"Angle"=492.0, "State"=FALSE}, {"Angle"=495.0, "State"=TRUE}, {"Angle"=498.0, "State"=FALSE}, {"Angle"=501.0, "State"=TRUE}, {"Angle"=504.0, "State"=FALSE}, {"Angle"=507.0, "State"=TRUE}, {"Angle"=510.0, "State"=FALSE}, {"Angle"=513.0, "State"=TRUE}, {"Angle"=516.0, "State"=FALSE}, {"Angle"=519.0, "State"=TRUE}, {"Angle"=522.0, "State"=FALSE}, {"Angle"=525.0, "State"=TRUE}, {"Angle"=528.0, "State"=FALSE}, {"Angle"=531.0, "State"=TRUE}, {"Angle"=534.0, "State"=FALSE}, {"Angle"=537.0, "State"=TRUE}, {"Angle"=540.0, "State"=FALSE}, {"Angle"=543.0, "State"=TRUE}, {"Angle"=546.0, "State"=FALSE}, {"Angle"=549.0, "State"=TRUE}, {"Angle"=552.0, "State"=FALSE}, {"Angle"=555.0, "State"=TRUE}, {"Angle"=558.0, "State"=FALSE}, {"Angle"=561.0, "State"=TRUE}, {"Angle"=564.0, "State"=FALSE}, {"Angle"=567.0, "State"=TRUE}, {"Angle"=570.0, "State"=FALSE}, {"Angle"=573.0, "State"=TRUE}, {"Angle"=576.0, "State"=FALSE}, {"Angle"=579.0, "State"=TRUE}, {"Angle"=582.0, "State"=FALSE}, {"Angle"=585.0, "State"=TRUE}, {"Angle"=588.0, "State"=FALSE}, {"Angle"=591.0, "State"=TRUE}, {"Angle"=594.0, "State"=FALSE}, {"Angle"=597.0, "State"=TRUE}, {"Angle"=600.0, "State"=FALSE}, {"Angle"=603.0, "State"=TRUE}, {"Angle"=606.0, "State"=FALSE}, {"Angle"=609.0, "State"=TRUE}, {"Angle"=612.0, "State"=FALSE}, {"Angle"=615.0, "State"=TRUE}, {"Angle"=618.0, "State"=FALSE}, {"Angle"=621.0, "State"=TRUE}, {"Angle"=624.0, "State"=FALSE}, {"Angle"=627.0, "State"=TRUE}, {"Angle"=630.0, "State"=FALSE}, {"Angle"=633.0, "State"=TRUE}, {"Angle"=636.0, "State"=FALSE}, {"Angle"=639.0, "State"=TRUE}, {"Angle"=642.0, "State"=FALSE}, {"Angle"=645.0, "State"=TRUE}, {"Angle"=648.0, "State"=FALSE}, {"Angle"=651.0, "State"=TRUE}, {"Angle"=654.0, "State"=FALSE}, {"Angle"=657.0, "State"=TRUE}, {"Angle"=660.0, "State"=FALSE}, {"Angle"=663.0, "State"=TRUE}, {"Angle"=666.0, "State"=FALSE}, {"Angle"=669.0, "State"=TRUE}, {"Angle"=672.0, "State"=FALSE}, {"Angle"=675.0, "State"=TRUE}, {"Angle"=678.0, "State"=FALSE}, {"Angle"=681.0, "State"=TRUE}, {"Angle"=684.0, "State"=FALSE}, {"Angle"=687.0, "State"=TRUE}, {"Angle"=690.0, "State"=FALSE}, {"Angle"=693.0, "State"=TRUE}, {"Angle"=696.0, "State"=FALSE}, {"Angle"=699.0, "State"=TRUE}, {"Angle"=702.0, "State"=FALSE}, {"Angle"=705.0, "State"=TRUE}], "Aux 1"=[{"Angle"=12.0, "State"=TRUE}, {"Angle"=24.0, "State"=FALSE}, {"Angle"=48.0, "State"=TRUE}, {"Angle"=60.0, "State"=FALSE}, {"Angle"=132.0, "State"=TRUE}, {"Angle"=144.0, "State"=FALSE}, {"Angle"=198.0, "State"=TRUE}, {"Angle"=252.0, "State"=TRUE}, {"Angle"=264.0, "State"=FALSE}, {"Angle"=318.0, "State"=TRUE}, {"Angle"=372.0, "State"=TRUE}, {"Angle"=384.0, "State"=FALSE}, {"Angle"=438.0, "State"=TRUE}, {"Angle"=492.0, "State"=TRUE}, {"Angle"=504.0, "State"=FALSE}, {"Angle"=558.0, "State"=TRUE}, {"Angle"=612.0, "State"=TRUE}, {"Angle"=624.0, "State"=FALSE}, {"Angle"=678.0, "State"=TRUE}], "Aux 2"=[{"Angle"=12.0, "State"=TRUE}, {"Angle"=24.0, "State"=FALSE}, {"Angle"=48.0, "State"=TRUE}, {"Angle"=60.0, "State"=FALSE}, {"Angle"=132.0, "State"=TRUE}, {"Angle"=144.0, "State"=FALSE}, {"Angle"=198.0, "State"=TRUE}, {"Angle"=252.0, "State"=TRUE}, {"Angle"=264.0, "State"=FALSE}, {"Angle"=318.0, "State"=TRUE}, {"Angle"=372.0, "State"=TRUE}, {"Angle"=384.0, "State"=FALSE}, {"Angle"=438.0, "State"=TRUE}, {"Angle"=492.0, "State"=TRUE}, {"Angle"=504.0, "State"=FALSE}, {"Angle"=558.0, "State"=TRUE}, {"Angle"=612.0, "State"=TRUE}, {"Angle"=624.0, "State"=FALSE}, {"Angle"=678.0, "State"=TRUE}], "Aux 3"=[], "Aux 4"=[]}  # EPTxPatternSettings
    }
  }
  n9 = call <vilib>:"time2ticks.vi"("Clock Frequency (MHz, 40)"=w10, "Time (msec)"=w36) -> ("Ticks"=w37:u32)
  n10 = call <vilib>:"time2ticks.vi"("Clock Frequency (MHz, 40)"=w10, "Time (msec)"=w35) -> ("Ticks"=w38:u32)
  n11 = call <vilib>:"time2ticks.vi"("Clock Frequency (MHz, 40)"=w10, "Time (msec)"=w34) -> ("Ticks"=w39:u32)
  n12 = call <vilib>:"time2ticks.vi"("Clock Frequency (MHz, 40)"=w10, "Time (msec)"=w33) -> ("Ticks"=w40:u32)
  n13 = call <vilib>:"time2ticks.vi"("Clock Frequency (MHz, 40)"=w10, "Time (msec)"=w32) -> ("Ticks"=w41:u32)
  n14 = case shown="True" w16 {
    tunnel: w15 -> [_ w150]
    tunnel: [w149 w150] -> w5
    tunnel: w8 -> [w149 _]
    frame False {
    }
    frame True {
      "AvgSpeed" <- w150
    }
  }
  n15 = call "EPTx_Patch1.0.vi"("Inj_Duration_in"="Inj_Duration_in", "DrvMode"=w28, "Adv_Speed"=w5, "Inj_Timing"="Inj_Timing") -> ("Inj_Timing_DBTDC"=w12:sgl, "Cmd_Duration"=w3:T20)  [unwired: 6 in]
  n16 = Unbundle By Name(w3) -> ("Duration1"=w55:sgl, "Duratiion2"=w54:sgl, "Duration3"=w53:sgl, "Duration4"=w52:sgl, "Duration5"=w51:sgl, "Duration6"=w50:sgl, "Duration7"=w49:sgl, "Duration8"=w48:sgl, "Duration9"=w47:sgl, "Duration10"=w46:sgl, "Duration11"=w45:sgl, "Duration12"=w44:sgl)
  n17 = Bundle(cluster=T20 {"Duration1"=0.0, "Duratiion2"=0.0, "Duration3"=0.0, "Duration4"=0.0, "Duration5"=0.0, "Duration6"=0.0, "Duration7"=0.0, "Duration8"=0.0, "Duration9"=0.0, "Duration10"=0.0, "Duration11"=0.0, "Duration12"=0.0} ("Cmd_Duration"), "Duration1"=w55, "Duratiion2"=w54, "Duration3"=w53, "Duration4"=w52, "Duration5"=w51, "Duration6"=w50, "Duration7"=w49, "Duration8"=w48, "Duration9"=w47, "Duration10"=w46, "Duration11"=w45, "Duration12"=w44) -> (w43:T20)
  n18 = Unbundle(w43) -> ("Duration1"=w94:sgl, "Duratiion2"=w87:sgl, "Duration3"=w86:sgl, "Duration4"=w85:sgl, "Duration5"=w84:sgl, "Duration6"=w83:sgl, "Duration7"=w82:sgl, "Duration8"=w81:sgl, "Duration9"=w67:sgl, "Duration10"=w66:sgl, "Duration11"=w61:sgl, "Duration12"=w60:sgl)
  n19 = To Single Precision Float(number=w5) -> (single precision float=w4:sgl)
  n20 = call <vilib>:"Time2CAD.vi"("Time [ms]"=w98, "Speed (RPM)"=w5) -> ("CAD"=w99:sgl)
  n21 = Add(x=w12, y=w99) -> (x+y=w100:sgl)
  n22 = call <vilib>:"Time2CAD.vi"("Time [ms]"=sgl 3.0, "Speed (RPM)"=w5) -> ("CAD"=w115:sgl)
  "CAD" <- w115
  n23 = call <vilib>:"CAD2Time.vi"("CAD"=w94, "Speed (RPM)"=w4) -> ("Time [ms]"=w97:sgl)
  n24 = call <vilib>:"CAD2Time.vi"("CAD"=w87, "Speed (RPM)"=w5) -> ("Time [ms]"=w95:sgl)
  n25 = call <vilib>:"CAD2Time.vi"("CAD"=w86, "Speed (RPM)"=w5) -> ("Time [ms]"=w93:sgl)
  n26 = call <vilib>:"CAD2Time.vi"("CAD"=w85, "Speed (RPM)"=w5) -> ("Time [ms]"=w92:sgl)
  n27 = call <vilib>:"CAD2Time.vi"("CAD"=w84, "Speed (RPM)"=w5) -> ("Time [ms]"=w88:sgl)
  n28 = call <vilib>:"CAD2Time.vi"("CAD"=w60, "Speed (RPM)"=w5) -> ("Time [ms]"=w62:sgl)
  n29 = call <vilib>:"CAD2Time.vi"("CAD"=w83, "Speed (RPM)"=w5) -> ("Time [ms]"=w89:sgl)
  n30 = call <vilib>:"CAD2Time.vi"("CAD"=w82, "Speed (RPM)"=w5) -> ("Time [ms]"=w90:sgl)
  n31 = call <vilib>:"CAD2Time.vi"("CAD"=w81, "Speed (RPM)"=w5) -> ("Time [ms]"=w91:sgl)
  n32 = call <vilib>:"CAD2Time.vi"("CAD"=w67, "Speed (RPM)"=w5) -> ("Time [ms]"=w69:sgl)
  n33 = call <vilib>:"CAD2Time.vi"("CAD"=w66, "Speed (RPM)"=w5) -> ("Time [ms]"=w68:sgl)
  n34 = call <vilib>:"CAD2Time.vi"("CAD"=w61, "Speed (RPM)"=w5) -> ("Time [ms]"=w63:sgl)
  n35 = call <vilib>:"time2ticks.vi"("Time (msec)"=w62) -> ("Ticks"=w58:u32)  [unwired: 1 in]
  n36 = call <vilib>:"time2ticks.vi"("Time (msec)"=w89) -> ("Ticks"=w73:u32)  [unwired: 1 in]
  n37 = call <vilib>:"time2ticks.vi"("Time (msec)"=w90) -> ("Ticks"=w72:u32)  [unwired: 1 in]
  n38 = call <vilib>:"time2ticks.vi"("Time (msec)"=w91) -> ("Ticks"=w71:u32)  [unwired: 1 in]
  n39 = call <vilib>:"time2ticks.vi"("Time (msec)"=w69) -> ("Ticks"=w65:u32)  [unwired: 1 in]
  n40 = call <vilib>:"time2ticks.vi"("Time (msec)"=w68) -> ("Ticks"=w64:u32)  [unwired: 1 in]
  n41 = call <vilib>:"time2ticks.vi"("Time (msec)"=w63) -> ("Ticks"=w59:u32)  [unwired: 1 in]
  n42 = call <vilib>:"time2ticks.vi"("Time (msec)"=w97) -> ("Ticks"=w78:u32)  [unwired: 1 in]
  n43 = call <vilib>:"time2ticks.vi"("Time (msec)"=w95) -> ("Ticks"=w77:u32)  [unwired: 1 in]
  n44 = call <vilib>:"time2ticks.vi"("Time (msec)"=w93) -> ("Ticks"=w76:u32)  [unwired: 1 in]
  n45 = call <vilib>:"time2ticks.vi"("Time (msec)"=w92) -> ("Ticks"=w75:u32)  [unwired: 1 in]
  n46 = call <vilib>:"time2ticks.vi"("Time (msec)"=w88) -> ("Ticks"=w74:u32)  [unwired: 1 in]
  n47 = call <vilib>:"Simulation Control.vi"("SimulatorConfig"="SimulatorConfig", "Frequency (40M) [Hz]"=w144) -> ("EPTxSimulatorConfig"=w57:T9, "Loading"=w1:bool)  [unwired: 12 in]
  n48 = call <vilib>:"EPTx - Core Control.vi"("EPTxSupervisor"="EPTxSupervisor_rt", "Load"=w141, "EPTxSettings"=w101, "EPTxState"="EPTxState", "Frequency (40M) [Hz]"=w144, "Stall Speed (200) [RPM]"=w134, "Filters (0)"="EPTxFilters", "History (63) [CAD]"=w135) -> ("EPTxConfig"=w137:T8, "EPTxControl"=→"EPTxControl":T3, "EPTxData"=→"EPTxData":T2, "Loading"=w2:bool)  [unwired: 3 in, 1 out]
  n49 = Replace Array Subset(array=w80, new element #1=w78, new element #2=w77, new element #3=w76, new element #4=w75, new element #5=w74, new element #6=w73, new element #7=w72, new element #8=w71, new element #9=w65, new element #10=w64, new element #11=w59, new element #12=w58) -> (w79:u32[])  [unwired: 12 in]
  n50 = call <vilib>:"Pattern Control.vi"("Load"=w141, "EPTxPatternSettings"=w143, "PatternConfig"="PatternConfig", "Frequency (40M) [Hz]"=w144) -> ("EPTxPatternConfig"=→"EPTxPatternConfig":T4, "Loading"=w139:bool)  [unwired: 10 in]
  n51 = Bundle By Name(cluster=w96, "DurationSeq"=w79, "CmdLevelSeq"=w6, "ContinueSeq"=w7) -> (→"Cmd_Seq":T19)
  n52 = Subtract(x=sgl 90.0 ("Cylinder TDC [Absolute CAD]"), y=w100) -> (x-y=w102:sgl)
  n53 = Subtract(x=sgl 690.0 ("Cylinder TDC [Absolute CAD]"), y=w100) -> (x-y=w123:sgl)
  n54 = Subtract(x=sgl 210.0 ("Cylinder TDC [Absolute CAD]"), y=w100) -> (x-y=w125:sgl)
  n55 = Bundle By Name(cluster=w138, "EPTxConfig"=w137, "EPTxSimulatorConfig"=w57) -> (→"Config_number":T10)
  n56 = Subtract(x=sgl 450.0 ("Cylinder TDC [Absolute CAD]"), y=w100) -> (x-y=w120:sgl)
  n57 = Subtract(x=sgl 330.0 ("Cylinder TDC [Absolute CAD]"), y=w100) -> (x-y=w103:sgl)
  n58 = Subtract(x=sgl 570.0 ("Cylinder TDC [Absolute CAD]"), y=w100) -> (x-y=w104:sgl)
  n59 = Bundle By Name(cluster=w140, "Pattern Loading"=w139, "Config Loading"=w2, "Sim Loading"=w1) -> (→"Lighting":T28)
  n60 = Add(x=w120, y=w115) -> (x+y=w121:sgl)
  n61 = Add(x=w125, y=w115) -> (x+y=w126:sgl)
  n62 = Add(x=w102, y=w115) -> (x+y=w118:sgl)
  n63 = Add(x=w123, y=w115) -> (x+y=w124:sgl)
  n64 = Add(x=w103, y=w115) -> (x+y=w117:sgl)
  n65 = Add(x=w104, y=w115) -> (x+y=w116:sgl)
  n66 = Bundle By Name(cluster=w130, "Cylinder4_H_R [CAD]"=w102, "Cylinder4_H_F [CAD]"=w118) -> (w107:T24)
  n67 = Bundle By Name(cluster=w133, "Cylinder1_H_R [CAD]"=w125, "Cylinder1_H_F [CAD]"=w126) -> (w110:T27)
  n68 = Bundle By Name(cluster=w132, "Cylinder2_H_R [CAD]"=w123, "Cylinder2_H_F [CAD]"=w124) -> (w109:T26)
  n69 = Bundle By Name(cluster=w131, "Cylinder3_H_R [CAD]"=w120, "Cylinder3_H_F [CAD]"=w121) -> (w108:T25)
  n70 = Bundle By Name(cluster=w129, "Cylinder5_H_R [CAD]"=w103, "Cylinder5_H_F [CAD]"=w117) -> (w106:T23)
  n71 = Bundle By Name(cluster=w128, "Cylinder6_H_R [CAD]"=w104, "Cylinder6_H_F [CAD]"=w116) -> (w105:T22)
  n72 = Bundle By Name(cluster=T1 {"Main_Inj_Duration[Ticks]"=0, "Pre_Inj_1_Duration[Ticks]"=0, "Pre_Inj_2_Duration[Ticks]"=0, "Pre_Inj_3_Duration[Ticks]"=0, "Pre_Inj_4_Duration[Ticks]"=0, "CANTtigger_AdvTime[Ticks]"=0} ("Tick_output"), "Main_Inj_Duration[Ticks]"=w37, "Pre_Inj_1_Duration[Ticks]"=w38, "Pre_Inj_2_Duration[Ticks]"=w39, "Pre_Inj_3_Duration[Ticks]"=w40, "Pre_Inj_4_Duration[Ticks]"=w41, "CANTtigger_AdvTime[Ticks]"=w42) -> (→"Tick_output":T1)
  n73 = Bundle By Name(cluster=w111, "CylinderSig_1"=w110, "CylinderSig_2"=w109, "CylinderSig_3"=w108, "CylinderSig_4"=w107, "CylinderSig_5"=w106, "CylinderSig_6"=w105) -> (→"CylinderSig":T21)
